vi "Chroma_PowerSupply_CurrentSetting.vi"(8 "错误输入（无错误）":errorcluster, 9 "CurrentMAXSetting":sgl, 11 "VISA资源名称":refnum<visa-resource-name>="COM1") -> (0 "错误输出":errorcluster, 3 "VISA资源名称输出":refnum<visa-resource-name>)   [LabVIEW 2012]
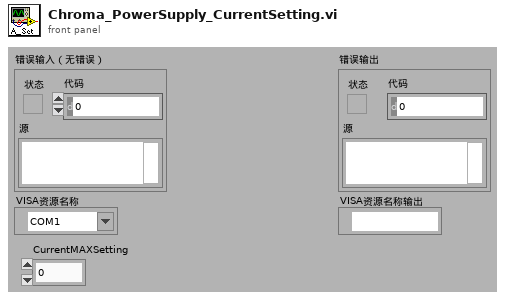
[diagram p1: front panel]
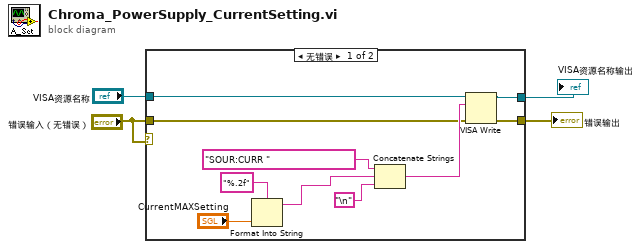
[diagram p0: block diagram]
diagram:
  n1 = case shown="无错误" "错误输入（无错误）" {
    tunnel: "VISA资源名称" -> [w12 w16]
    tunnel: "错误输入（无错误）" -> [w11 w15]
    tunnel: [w10 w16] -> w3
    tunnel: [w9 w15] -> w2
    frame No Error {
      n2 = Format Into String(format string="%.2f" ("格式字符串"), "CurrentMAXSetting") -> (resulting string=w5:string)  [unwired: 2 in, 1 out]
      n3 = Concatenate Strings("SOUR:CURR ", w5, "\n") -> (w13:string)
      n4 = VISA Write(VISA resource name=w12, write buffer=w13, error in (no error)=w11) -> (VISA resource name out=w10:refnum<visa-resource-name>, error out=w9:errorcluster)  [unwired: 1 out]
    }
    frame Error {
    }
  }
  "错误输出" <- w2
  "VISA资源名称输出" <- w3
